vi "Process Beacon.vi"(0 "Known Hosts in":T1[](array[typedef]), 7 "DiscoveredHost":T1={"Beacon"={"name"="", "addr"="", "port"=0, "ver"=10001}, "Last Seen"=timestamp(0 s since 1904-01-01)}) -> (4 "Known Hosts out":T1[](array[typedef]), 8 "Beacon Result":T3)   [LabVIEW 2020, in "epl-network.lvlib"]
uses:
  epl-network.lvlib
  Public/Discovery/Typedefs/Beacon Result.ctl
  Discovered Host.ctl
  Public/Discovery/Typedefs/Server Beacon.ctl
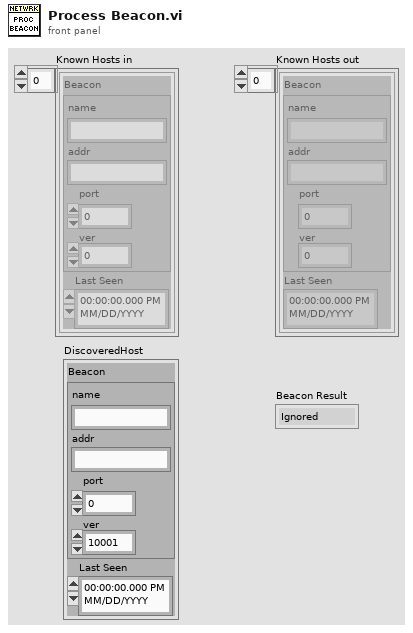
[diagram p1: front panel]
types:
  T1 = typedef "epl-network.lvlib/Discovered Host.ctl" = cluster{"Beacon":T2, "Last Seen":timestamp}
  T2 = typedef "epl-network.lvlib/Server Beacon.ctl" = cluster{"name":string, "addr":string, "port":u16, "ver":u16}
  T3 = typedef "epl-network.lvlib/Beacon Result.ctl" = enum16{"Ignored", "Updated", "Added"}
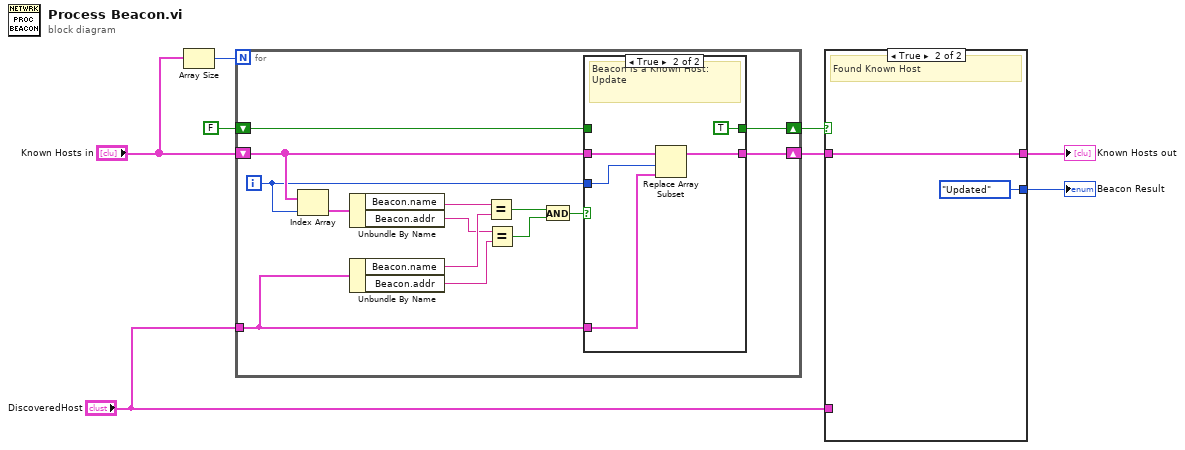
[diagram p0: block diagram]
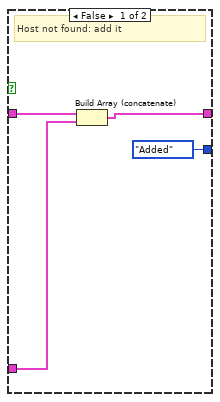
[diagram p2: hidden frame]
diagram:
  n1 = Array Size(array="Known Hosts in") -> (size(s)=w3:i32)
  n2 = for {
    N: w3 -> [_]
    tunnel: "DiscoveredHost" -> [w18]
    shift-right: [w10] -> w1
    shift-left: FALSE -> [w11]
    shift-right: [w17] -> w8
    shift-left: "Known Hosts in" -> [w13]
    i -> [w9]
    n3 = Index Array(array=w13, index=w9) -> (element=w12:T1)
    n4 = Unbundle By Name(w12) -> ("Beacon.name"=w22:string, "Beacon.addr"=w20:string)
    n5 = Unbundle By Name(w18) -> ("Beacon.name"=w21:string, "Beacon.addr"=w19:string)
    n6 = Equal?(x=w22, y=w21) -> (x = y?=w16:bool)
    n7 = Equal?(x=w20, y=w19) -> (x = y?=w15:bool)
    n8 = And(x=w16, y=w15) -> (x .and. y?=w14:bool)
    n9 = case shown="True" w14 {
      tunnel: w13 -> [w24 w28]
      tunnel: w18 -> [_ w25]
      tunnel: [w24 w27] -> w17
      tunnel: w11 -> [w23 _]
      tunnel: [w23 TRUE] -> w10
      tunnel: w9 -> [_ w26]
      frame False {
      }
      frame True {
        # "Beacon is a Known Host:\nUpdate"
        n10 = Replace Array Subset(array=w28, new element=w25, index=w26) -> (w27:T1[])
      }
    }
  }
  n11 = case shown="True" w1 {
    tunnel: w8 -> [w33 w35]
    tunnel: [w31 w35] -> w6
    tunnel: "DiscoveredHost" -> [w32 _]
    tunnel: [Beacon_Result."Added" ("Beacon Result") Beacon_Result."Updated" ("Beacon Result")] -> w5
    frame False {
      # "Host not found: add it"
      n12 = Build Array (concatenate)(w33, w32) -> (w31:T1[])
    }
    frame True {
      # "Found Known Host"
    }
  }
  "Beacon Result" <- w5
  "Known Hosts out" <- w6
